vi "Loop Period.vi"() -> (0 "dt":dbl)   [LabVIEW 2021]
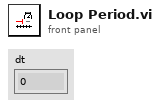
[diagram p1: front panel]
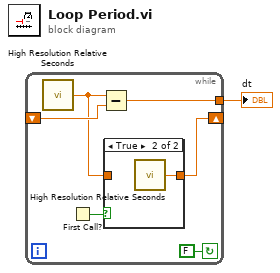
[diagram p0: block diagram]
diagram:
  n1 = while {
    shift-right: [w4] -> _
    shift-left: _ -> [w7]
    tunnel: [w6] -> w1
    stop <- FALSE continue-if-true
    n2 = call <vilib>:"High Resolution Relative Seconds.vi"() -> ("relative seconds"=w3:dbl)
    n3 = First Call?() -> (First Call?: T/F=w5:bool)
    n4 = Subtract(x=w3, y=w7) -> (x-y=w6:dbl)
    n5 = case shown="True" w5 {
      tunnel: [w8 w9] -> w4
      tunnel: w3 -> [w8 _]
      frame False {
      }
      frame True {
        n6 = call <vilib>:"High Resolution Relative Seconds.vi"() -> ("relative seconds"=w9:dbl)
      }
    }
  }
  "dt" <- w1
